vi "get hex string before separator.vi"(4 "Convert to hex?":bool=TRUE, 8 "error in (no error)":errorcluster={"status"=FALSE, "code"=0, "source"="No Error."}, 10 "String In":string, 11 "Separator In":i32) -> (0 "error out":errorcluster, 1 "after match out":string, 2 "hexadecimal 1 out":u32 format="0x%02x", 3 "hexadecimal string out":string, 5 "String Before and Separator":string)   [LabVIEW 2016]
panel:
  out "before match out":string
  out "length":i32
  out "unsigned byte array":u8[](array[numeric])
  out "whole match":string
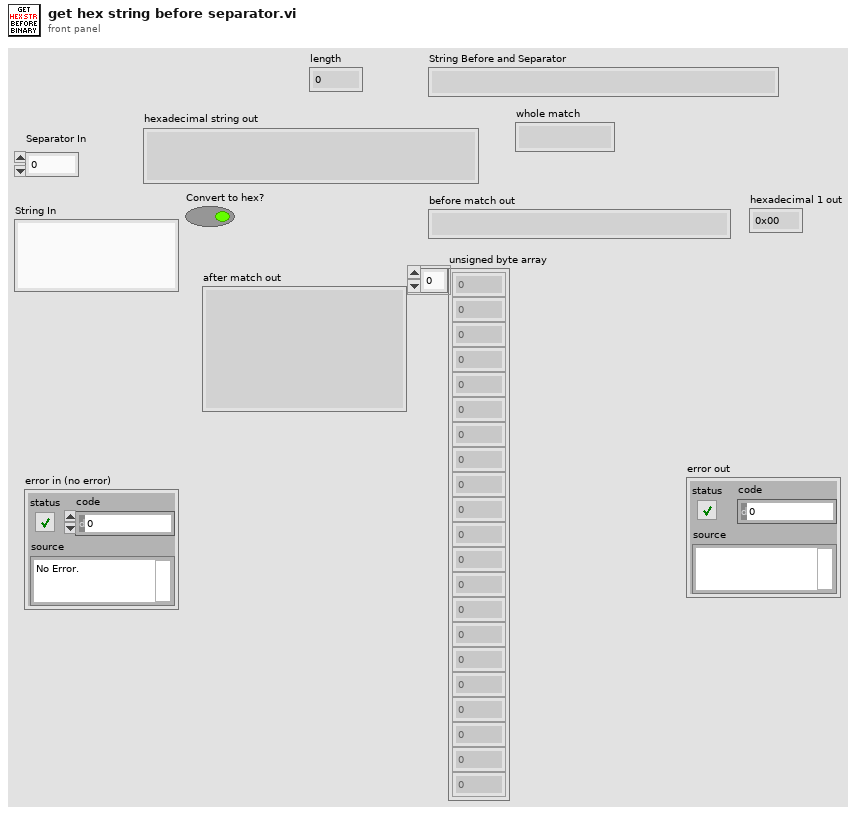
[diagram p1: front panel]
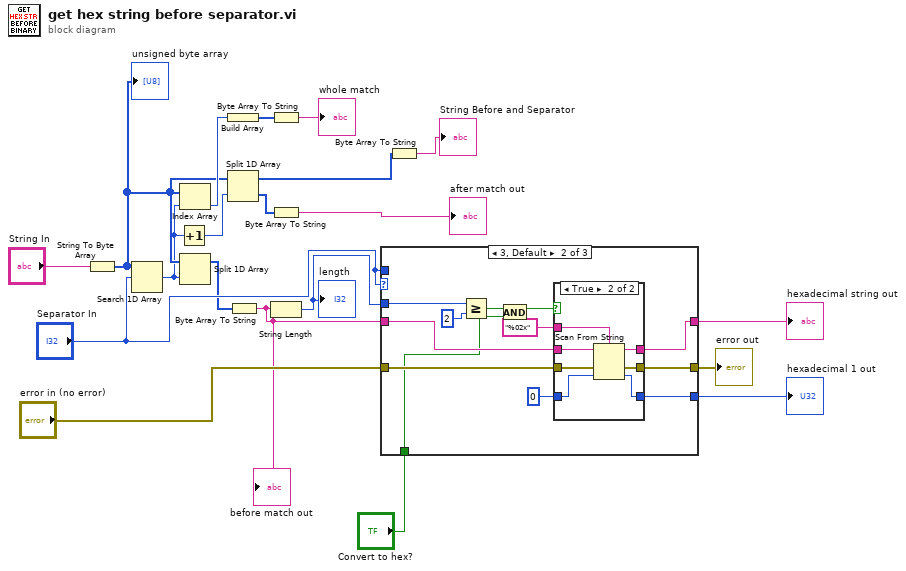
[diagram p0: block diagram]
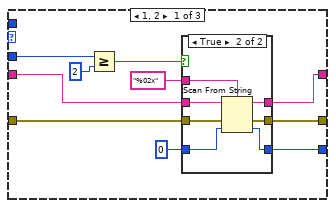
[diagram p2: hidden frame]
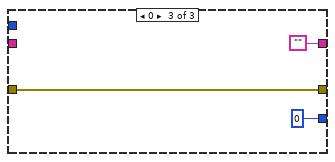
[diagram p5: hidden frame]
diagram:
  n1 = String To Byte Array(string="String In") -> (unsigned byte array=w6:u8[])
  "unsigned byte array" <- w6
  n2 = Search 1D Array(1D array=w6, element="Separator In") -> (index of element=w5:i32)  [unwired: 1 in]
  n3 = Increment(x=w5) -> (x+1=w16:i32)
  n4 = Index Array(array=w6, index=w5) -> (element=w12:u8)
  n5 = Split 1D Array(array=w6, index=w5) -> (first subarray=w4:u8[])  [unwired: 1 out]
  n6 = Build Array(w12) -> (w11:u8[])
  n7 = Split 1D Array(array=w6, index=w16) -> (first subarray=w2:u8[], second subarray=w15:u8[])
  n8 = Byte Array To String(unsigned byte array=w4) -> (string=w3:string)
  "before match out" <- w3
  n9 = Byte Array To String(unsigned byte array=w11) -> (string=→"whole match":string)
  n10 = Byte Array To String(unsigned byte array=w15) -> (string=→"after match out":string)
  n11 = String Length(string=w3) -> (length=w9:i32)
  "length" <- w9
  n12 = case shown="3, Default" "Separator In" {
    tunnel: [w30 w52 0] -> w20
    tunnel: [w28 w50 w65] -> w19
    tunnel: "error in (no error)" -> [w27 w49 w65]
    tunnel: "Separator In" -> [_ _ _]
    tunnel: w3 -> [w26 w48 _]
    tunnel: w9 -> [w23 w45 _]
    tunnel: [w21 w43 ""] -> w7
    tunnel: "Convert to hex?" -> [_ w41 _]
    frame 1, 2 {
      n13 = Greater Or Equal?(x=w23, y=2 ("x")) -> (x >= y?=w25:bool)
      n14 = case shown="True" w25 {
        tunnel: [w32 w40] -> w30
        tunnel: "%02x" ("format string") -> [_ w39]
        tunnel: [w33 w38] -> w28
        tunnel: w27 -> [w33 w37]
        tunnel: w26 -> [w31 w36]
        tunnel: 0 -> [w32 w35]
        tunnel: [w31 w34] -> w21
        frame False {
        }
        frame True {
          n15 = Scan From String(format string=w39, input string=w36, error in=w37, default 1=w35) -> (remaining string=w34:string, error out=w38:errorcluster, output 1=w40:i32)  [unwired: 1 in, 1 out]
        }
      }
    }
    frame 3, Default {
      n16 = Greater Or Equal?(x=w45, y=2 ("x")) -> (x >= y?=w47:bool)
      n17 = And(x=w47, y=w41) -> (x .and. y?=w42:bool)
      n18 = case shown="True" w42 {
        tunnel: [w54 w62] -> w52
        tunnel: "%02x" ("format string") -> [_ w61]
        tunnel: [w55 w60] -> w50
        tunnel: w49 -> [w55 w59]
        tunnel: w48 -> [w53 w58]
        tunnel: 0 -> [w54 w57]
        tunnel: [w53 w56] -> w43
        frame False {
        }
        frame True {
          n19 = Scan From String(format string=w61, input string=w58, error in=w59, default 1=w57) -> (remaining string=w56:string, error out=w60:errorcluster, output 1=w62:i32)  [unwired: 1 in, 1 out]
        }
      }
    }
    frame 0 {
    }
  }
  "hexadecimal string out" <- w7
  "hexadecimal 1 out" <- w20
  "error out" <- w19
  n20 = Byte Array To String(unsigned byte array=w2) -> (string=→"String Before and Separator":string)
